vi "Get Page VI.vi"(8 "error in (no error)":errorcluster, 9 "GUID":string, 10 "Item Ref":T1 format="%.0x", 11 "System Explorer Dispatcher in":refnum<class "System Explorer Dispatcher.lvclass">) -> (0 "error out":errorcluster, 2 "page reference":refnum<vi>, 3 "System Explorer Dispatcher out":refnum<class "System Explorer Dispatcher.lvclass">)   [LabVIEW 2020, in "Ballard ARINC 429 System Explorer.lvlib" / "Interfaces.lvlib" / "System Explorer Dispatcher.lvclass"]
uses:
  System Explorer Dispatcher.lvclass
  <vilib>/NI VeriStand/Custom Device API/Custom Device Item Ref.ctl
  <vilib>/NI VeriStand/Custom Device API/Custom Device API.lvlib
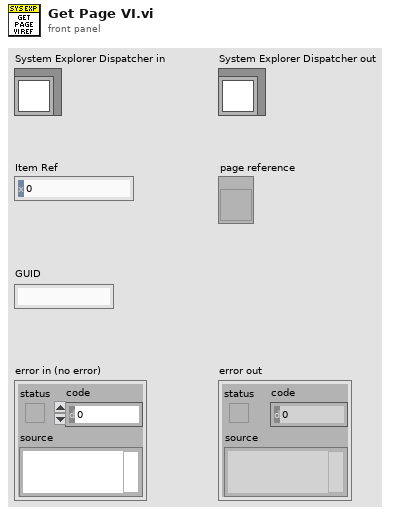
[diagram p1: front panel]
types:
  T1 = typedef "Custom Device API.lvlib/Custom Device Item Ref.ctl" = u64
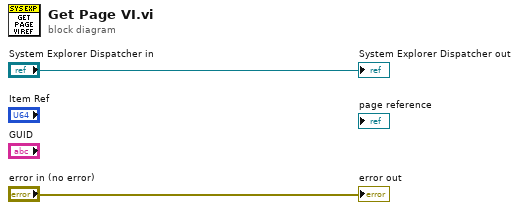
[diagram p0: block diagram]
diagram:
  "error out" <- "error in (no error)"
  "System Explorer Dispatcher out" <- "System Explorer Dispatcher in"
